vi "Get Bytes.vi"(11 "MsgPackArray in":refnum<class "MsgPackArray.lvclass">) -> (2 "Array":u8[](array[numeric]), 3 "MsgPackArray out":refnum<class "MsgPackArray.lvclass">)   [LabVIEW 2020, in "wamplv.lvlib" / "MsgPackArray.lvclass"]
uses:
  MsgPackArray.lvclass
  MsgPackArray.lvclass/MsgPackArray.ctl
  MessagePack/Format bytes.ctl
  MessagePack/MessagePack.lvclass
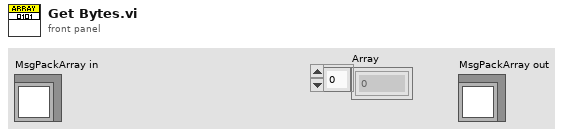
[diagram p1: front panel]
types:
  T1 = typedef "wamplv.lvlib/MsgPackArray.lvclass/Element.ctl" = cluster{"element bytes":u8[]}
  T2 = typedef "wamplv.lvlib/MessagePack.lvclass/Format bytes.ctl" = u8
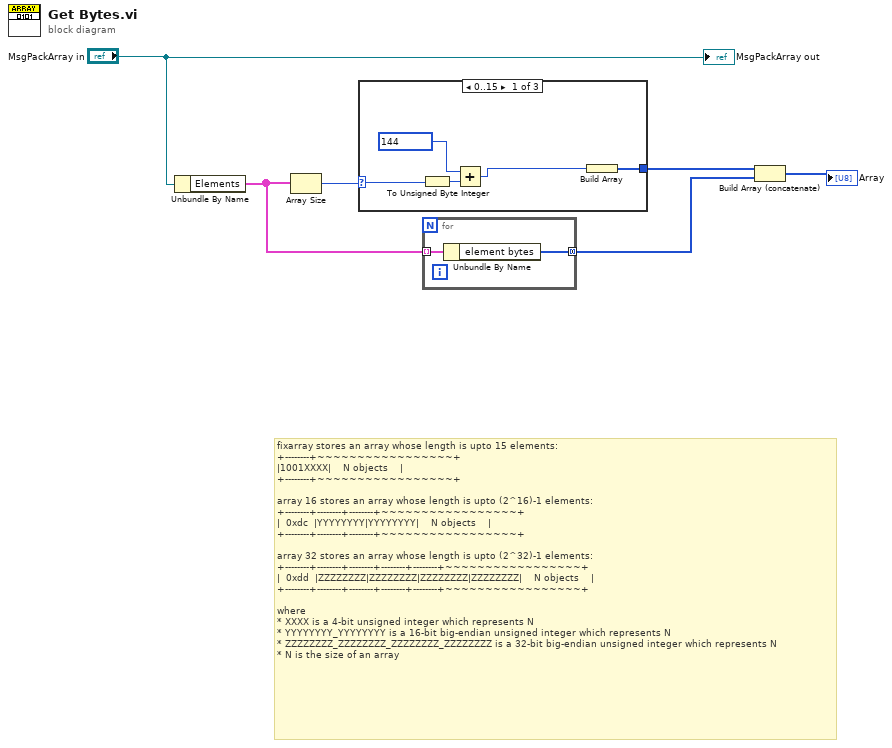
[diagram p0: block diagram]
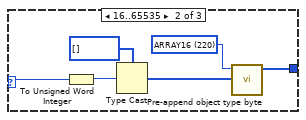
[diagram p2: hidden frame]
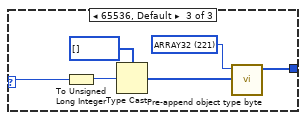
[diagram p3: hidden frame]
diagram:
  # "fixarray stores an array whose length is upto 15 elements:\n+--------+~~~~~~~~~~~~~~~~~+\n|1001XXXX|    N objects    |\n+--------+~~~~~~~~~~~~~~~~~+\n\narray 16 stores an array whose length is upto (2^16)-1 elements:\n+--------+--------+--------+~~~~~~~~~~~~~~~~~+\n|  0xdc  |YYYYYYYY|YYYYYYYY|    N objects    |\n+--------+--------+--------+~~~~~~~~~~~~~~~~~+\n\narray 32 stores an array whose length is upto (2^32)-1 elements:\n+--------+--------+--------+--------+--------+~~~~~~~~~~~~~~~~~+\n|  0xdd  |ZZZZZZZZ|ZZZZZZZZ|ZZZZZZZZ|ZZZZZZZZ|    N objects    |\n+--------+--------+--------+--------+--------+~~~~~~~~~~~~~~~~~+\n\nwhere\n* XXXX is a 4-bit unsigned integer which represents N\n* YYYYYYYY_YYYYYYYY is a 16-bit big-endian unsigned integer which represents N\n* ZZZZZZZZ_ZZZZZZZZ_ZZZZZZZZ_ZZZZZZZZ is a 32-bit big-endian unsigned integer which represents N\n* N is the size of an array"
  n1 = Unbundle By Name("MsgPackArray in") -> ("Elements"=w2:T1[])
  n2 = Array Size(array=w2) -> (size(s)=w3:i32)
  n3 = case shown="0..15" w3 {
    selector: w3 -> [w10 w17 w23]
    tunnel: [w8 w12 w18] -> w5
    frame 0..15 {
      n4 = To Unsigned Byte Integer(number=w10) -> (unsigned 8bit integer=w9:u8)
      n5 = Add(x=u8 144 ("y"), y=w9) -> (x+y=w7:u8)
      n6 = Build Array(w7) -> (w8:u8[])
    }
    frame 16..65535 {
      w13 = T2 220 items=["nil"=192, "UINT8"=204, "UINT16"=205, "UINT32"=206, "UINT64"=207, "INT8"=208, "INT16"=209, "INT32"=210, "INT64"=211, "FALSE"=194, "TRUE"=195, "SGL"=202, "DBL"=203, "ARRAY16"=220, "ARRAY32"=221] ("Format byte")
      n7 = To Unsigned Word Integer(number=w17) -> (unsigned 16bit integer=w15:u16)
      n8 = Type Cast(type=u8[] [] ("bytes"), x=w15) -> (*(type *) &x=w14:u8[])
      n9 = call "Pre-append object type byte.vi"("data in"=w14, "Format byte"=w13) -> ("bytes add"=w12:u8[])  [unwired: 9 in]
    }
    frame 65536, Default {
      w19 = T2 221 items=["nil"=192, "UINT8"=204, "UINT16"=205, "UINT32"=206, "UINT64"=207, "INT8"=208, "INT16"=209, "INT32"=210, "INT64"=211, "FALSE"=194, "TRUE"=195, "SGL"=202, "DBL"=203, "ARRAY16"=220, "ARRAY32"=221] ("Format byte")
      n10 = To Unsigned Long Integer(number=w23) -> (unsigned 32bit integer=w21:u32)
      n11 = Type Cast(type=u8[] [] ("bytes"), x=w21) -> (*(type *) &x=w20:u8[])
      n12 = call "Pre-append object type byte.vi"("data in"=w20, "Format byte"=w19) -> ("bytes add"=w18:u8[])  [unwired: 9 in]
    }
  }
  n13 = for {
    tunnel: w2 -> [w25] mode=indexing
    tunnel: [w24] -> w1 mode=concatenating
    n14 = Unbundle By Name(w25) -> ("element bytes"=w24:u8[])
  }
  n15 = Build Array (concatenate)(w5, w1) -> (→"Array":u8[])
  "MsgPackArray out" <- "MsgPackArray in"
